vi "FPGA Start Sample.vi"(11 "Sample Period (uSec)":u32) -> (0 "error out":errorcluster)   [LabVIEW 2014]
uses:
  <vilib>/rvi/eio/common/nirviEmuClasses.ctl
  <vilib>/rvi/Emulation/niFpgaGetClockAttributes.vi
  <vilib>/rvi/Emulation/niFpgaSctlEmulationGetInTimedLoop.vi
  <vilib>/rvi/Emulation/niFpgaEmulationReportErrorSimple.vi
  FPGA Globals.vi
  <vilib>/rvi/eio/common/nirviEmuTemplateMethod_errors.vi
  <vilib>/rvi/Emulation/niFpgaProcessEmulError.vi
  <vilib>/rvi/Emulation/niFpgaCriticalErrorInLSC.vi
  <vilib>/eio/EIOGrowableMethodNode/genericMethod/EIOGrowableMethodNode.xnode
  <vilib>/rvi/eio/nirviEIOMethodImplementation/nirviEIOMethodImplementation.xnode
  <vilib>/rvi/eio/nirviErrorMerge/nirviErrorMerge.xnode
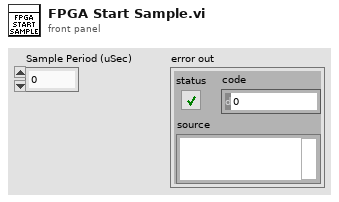
[diagram p1: front panel]
types:
  T1 = typedef "nirviEmuClasses.ctl" = enum16{"IO Read", "IO Write", "Method", "Property Read", "Property Write"}
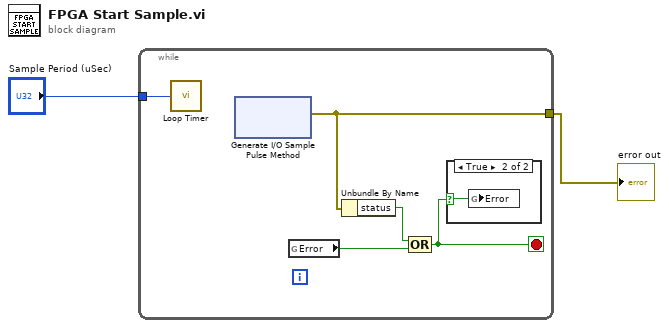
[diagram p0: block diagram]
diagram:
  n1 = while {
    tunnel: "Sample Period (uSec)" -> [w7]
    tunnel: [w5] -> w2
    stop <- w4 stop-if-true
    n2 = call "Loop Timer"("Count(uSec)"=w7) -> ()  [unwired: 1 out]
    n3 = xnode "Generate I/O Sample Pulse Method"() -> ("error out"=w5:errorcluster)  [unwired: 2 in, 1 out]
    n4 = global read "FPGA Globals.vi" "Error"() -> (w3:bool)
    n5 = Unbundle By Name(w5) -> ("status"=w6:bool)
    n6 = Compound Arithmetic op=OR(w6, w3) -> (w4:bool)
    n7 = case shown="True" w4 {
      selector: w4 -> [_ w52]
      frame False {
      }
      frame True {
        n8 = global write "FPGA Globals.vi" "Error"(w52) -> ()
      }
    }
  }
  "error out" <- w2
